vi "write_attributes.vi"(8 "error in (no error)":errorcluster, 10 "attributes":T1, 11 "GradientBoostingRegressor in":refnum<class "GradientBoostingRegressor.lvclass">) -> (0 "error out":errorcluster, 3 "GradientBoostingRegressor out":refnum<class "GradientBoostingRegressor.lvclass">)   [LabVIEW 2020, in "GradientBoostingRegressor.lvclass"]
uses:
  GradientBoostingRegressor.lvclass
  Controls/gradient_boosting_regressor_attributes.ctl
  GradientBoostingRegressor.lvclass/GradientBoostingRegressor.ctl
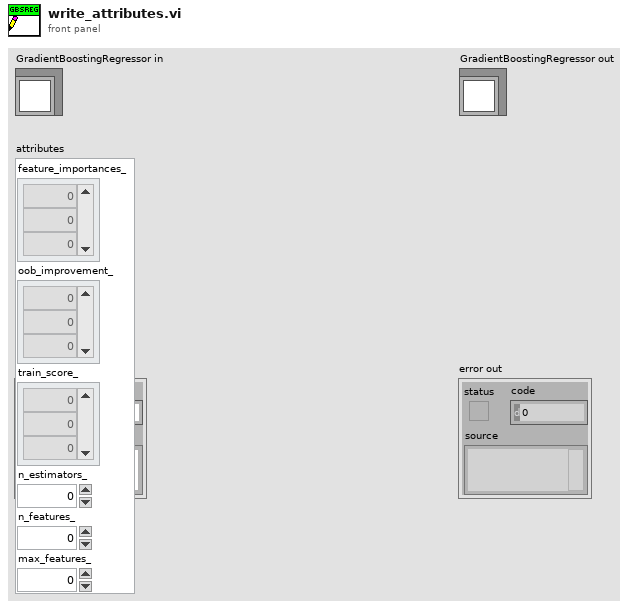
[diagram p1: front panel]
types:
  T1 = typedef "gradient_boosting_regressor_attributes.ctl" = cluster{"feature_importances_":dbl[], "oob_improvement_":dbl[], "train_score_":dbl[], "n_estimators_":dbl, "n_features_":dbl, "max_features_":dbl}
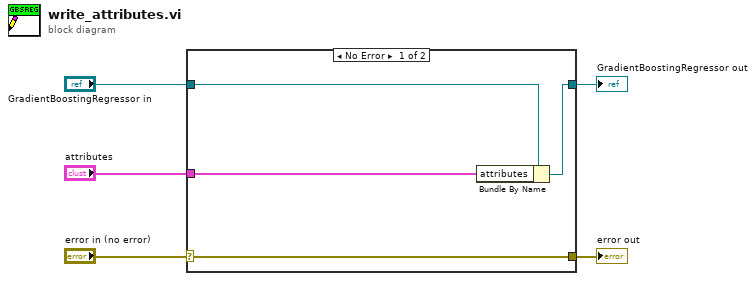
[diagram p0: block diagram]
diagram:
  n1 = case shown="No Error" "error in (no error)" {
    selector: "error in (no error)" -> [w9 w10]
    tunnel: [w9 w10] -> w4
    tunnel: [w7 w11] -> w2
    tunnel: "GradientBoostingRegressor in" -> [w8 w11]
    tunnel: "attributes" -> [w6 _]
    frame No Error {
      n2 = Bundle By Name(cluster=w8, "attributes"=w6) -> (w7:refnum<class "GradientBoostingRegressor.lvclass">)
    }
    frame Error {
    }
  }
  "error out" <- w4
  "GradientBoostingRegressor out" <- w2
